vi "test - List CSM Modules.vi"(8 "error in (no error)":errorcluster, 11 "TestCase in":refnum<class "testcase-Basic-Function.lvclass">) -> (0 "error out":errorcluster, 3 "TestCase out":refnum<class "testcase-Basic-Function.lvclass">)   [LabVIEW 2017, in "testcase-Basic-Function.lvclass"]
uses:
  testcase-Basic-Function.lvclass
  testcase-Basic-Function.lvclass/testcase-Basic-Function.ctl
  user.lib/_NEVSTOP/Communicable State Machine(CSM)/_Support/FGV-BroadcastRegistry/global-CSMQ FGV Change Flag.vi
  user.lib/_NEVSTOP/Communicable State Machine(CSM)/_Support/CSMQ/_CSMOFGV.vi
  <vilib>/addons/_JKI Toolkits/VI Tester/TestCase.llb/TestCase.lvclass
  user.lib/_NEVSTOP/Communicable State Machine(CSM)/Communicable State Machine.lvlib
  C:/Program Files (x86)/National Instruments/LabVIEW 2017/vi.lib/addons/_JKI Toolkits/VI Tester/TestCase.llb/TestCase.lvclass
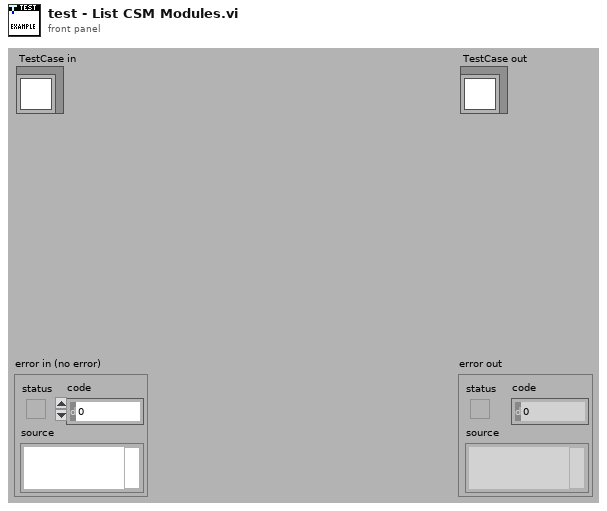
[diagram p1: front panel]
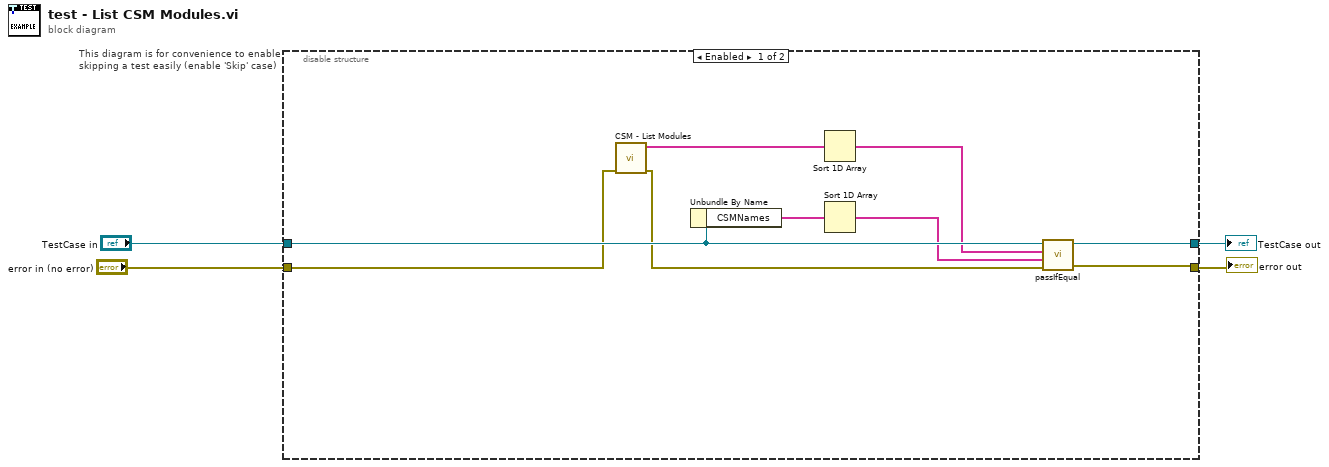
[diagram p0: block diagram]
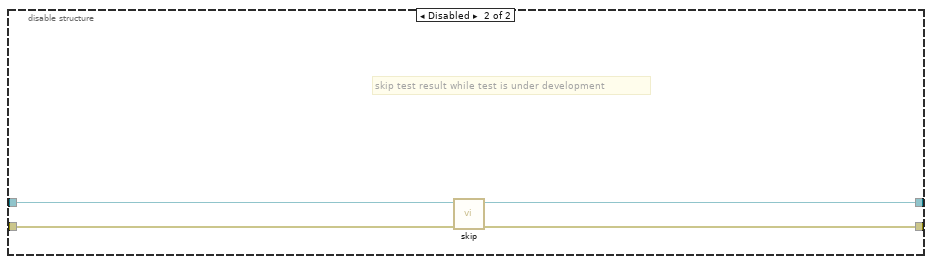
[diagram p2: hidden frame]
diagram:
  n1 = disable-structure "This diagram is for convenience to enable skipping a test easily (enable 'Skip' case)" shown="Enabled" {
    disable-tunnel: "TestCase in" -> [w10 w17]
    disable-tunnel: [w13 w15] -> w1
    disable-tunnel: [w12 w16] -> w3
    disable-tunnel: "error in (no error)" -> [w9 w14]
    frame Enabled {
      n2 = call "CSM - List Modules.vi"("Error in"=w9) -> ("Error out"=w8:errorcluster, "Module Names"=w11:string[])  [unwired: 9 in]
      n3 = Unbundle By Name(w10) -> ("CSMNames"=w7:string[])
      n4 = Sort 1D Array(array=w11) -> (sorted array=w6:string[])
      n5 = Sort 1D Array(array=w7) -> (sorted array=w5:string[])
      n6 = call-dynamic "passIfEqual.vi"("error in (no error)"=w8, "y"=w5, "x"=w6, "TestCase in"=w10) -> ("error out"=w12:errorcluster, "TestCase out"=w13:refnum<class "testcase-Basic-Function.lvclass">)  [unwired: 6 in]
    }
    frame Disabled {
      # "skip test result while test is under development"
      n7 = call <vilib>:"skip.vi"("error in (no error)"=w14, "TestCase in"=w17) -> ("error out"=w16:errorcluster, "TestCase out"=w15:refnum<class "testcase-Basic-Function.lvclass">)  [unwired: 8 in]
    }
  }
  "error out" <- w3
  "TestCase out" <- w1
